vi "GLOBAL Sub-Frames.vi"() -> ()   [LabVIEW 2015]
panel:
  in  "Sub-Frames":u16[][][](array[numeric])
  # "NOTE:\nThis global variable contains the current array of sub-frames.\nIt belongs to the 'Virtual Camera' class and should only ever\nbe written to by physical cameras that are part of a virtual\ncamera, and each of them may only access the sub-frame\ncorresponding to their initialization number."
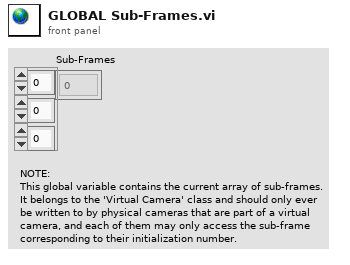
[diagram p1: front panel]
diagram:
